vi "Display Tree Item.vi"(8 "error in (no error)":errorcluster, 10 "Tag":string, 11 "Application Data in":T1) -> (0 "error out":errorcluster, 3 "Application Data out":T1)   [LabVIEW 2017, in "DSF Mini Explorer.lvlib"]
uses:
  DSF Mini Explorer.lvlib
  Application Data.ctl
  VeriStand/Data Sharing Custom Device/Source/DSF Core.lvlibp/Classes/Configuration/Configuration Session.lvclass
  View Mode.ctl
  VeriStand/Data Sharing Custom Device/Source/DSF Core.lvlibp/Classes/Configuration/Read Plugin.vi
  VeriStand/Data Sharing Custom Device/Source/DSF Core.lvlibp/Classes/Configuration/Read Settings.vi
  VeriStand/Data Sharing Custom Device/Source/DSF Core.lvlibp/Classes/Configuration/Read Channel.vi
  VeriStand/Data Sharing Custom Device/Source/DSF Core.lvlibp/Classes/Configuration/Read Transfer.vi
  VeriStand/Data Sharing Custom Device/Source/DSF Core.lvlibp/Classes/Configuration/Read Group.vi
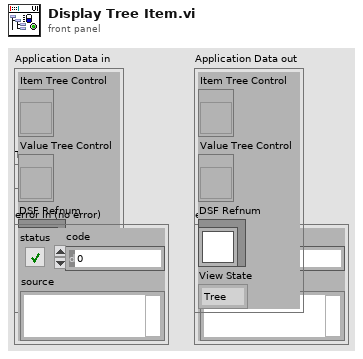
[diagram p1: front panel]
types:
  T1 = typedef "DSF Mini Explorer.lvlib/Application Data.ctl" = cluster{"Item Tree Control":refnum<vi>, "Value Tree Control":refnum<vi>, "DSF Refnum":refnum<class "Configuration Session.lvclass">, "View State":T2}
  T2 = typedef "DSF Mini Explorer.lvlib/View Mode.ctl" = enum16{"Tree", "List"}
  T3 = typedef "DSF Core.lvlibp/DSF Version Info.ctl" = cluster{"major":u32, "minor":u32, "fix":u32, "build":string}
  T4 = typedef "DSF Mini Explorer.lvlib/Tree Item Type.ctl" = enum16{"Plugin", "Group", "Transfer", "Channel", "Setting"}
  T5 = typedef "DSF Core.lvlibp/DSF Group Info.ctl" = cluster{"direction":T6, "timing":T7, "transfer ids":string[], "settings id":string, "thread":i32, "timeout behavior":T8}
  T6 = typedef "DSF Core.lvlibp/DSF Direction.ctl" = enum8{"Tx", "Rx"}
  T7 = typedef "DSF Core.lvlibp/DSF Timing Info.ctl" = cluster{"priority":u64, "decimation":u64, "offset":u64}
  T8 = typedef "DSF Core.lvlibp/DSF Timeout Behavior.ctl" = enum8{"Increment Late Count", "Throw Error"}
  T9 = typedef "DSF Core.lvlibp/DSF Transfer Info.ctl" = cluster{"byte order":T10, "channel ids":string[], "settings id":string}
  T10 = typedef "DSF Core.lvlibp/DSF Byte Order.ctl" = enum8{"big-endian", "little-endian"}
  T11 = typedef "DSF Core.lvlibp/DSF Channel Info.ctl" = cluster{"string buffer offset":u64, "string data type":T12, "engine data type":T12, "settings id":string, "units":string}
  T12 = typedef "DSF Core.lvlibp/DSF Data Type.ctl" = enum8{"Bool", "SGL", "DBL", "I8", "I16", "I32", "I64", "U8", "U16", "U32", "U64"}
  T13 = typedef "DSF Core.lvlibp/DSF Settings Info.ctl" = cluster{"key":string, "value":string}[]
  T14 = typedef "DSF Core.lvlibp/DSF Plugin Info.ctl" = cluster{"components":string[], "timing":T7, "group ids":string[], "settings id":string, "threads":T15[]}
  T15 = typedef "DSF Core.lvlibp/DSF Engine Plugin Thread Configuration.ctl" = cluster{"buffer converter settings":T13, "transceiver settings":T13, "custom settings":T13, "processor":i32, "priority offset":i16}
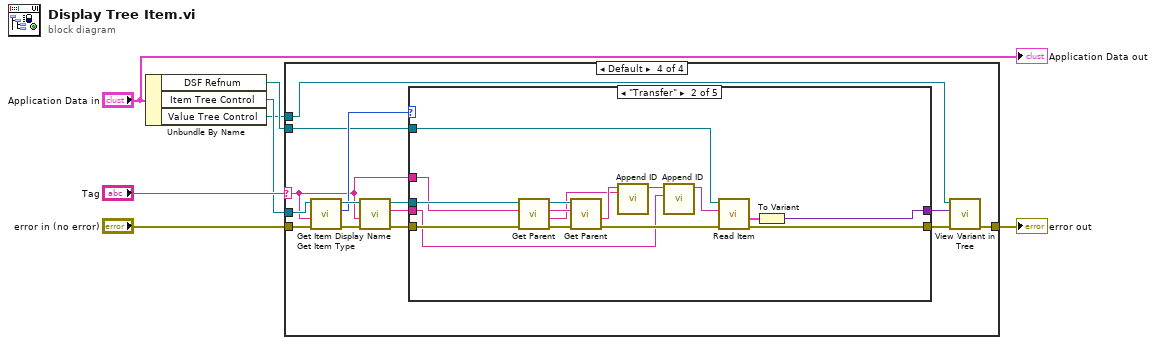
[diagram p0: block diagram]
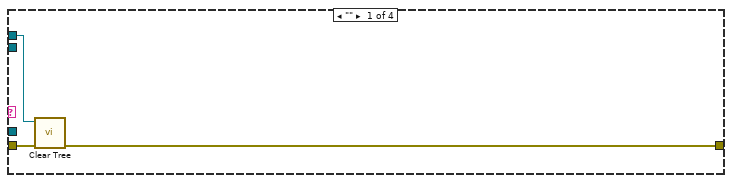
[diagram p2: hidden frame]
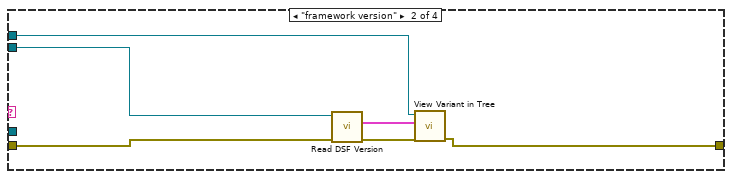
[diagram p3: hidden frame]
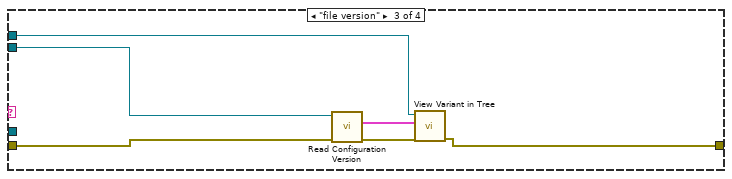
[diagram p4: hidden frame]
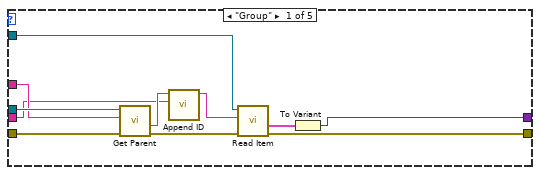
[diagram p5: hidden frame]
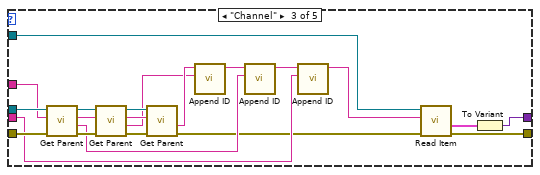
[diagram p6: hidden frame]
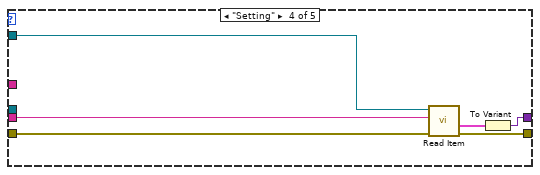
[diagram p7: hidden frame]
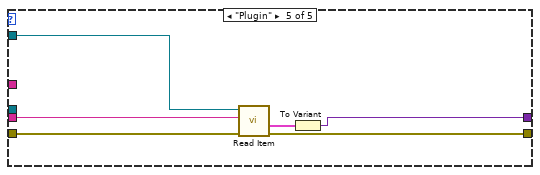
[diagram p8: hidden frame]
diagram:
  n1 = Unbundle By Name("Application Data in") -> ("DSF Refnum"=w5:refnum<class "Configuration Session.lvclass">, "Item Tree Control"=w4:refnum<vi>, "Value Tree Control"=w2:refnum<vi>)
  n2 = case shown="Default" "Tag" {
    selector: "Tag" -> [_ _ _ w24]
    tunnel: w5 -> [_ w16 w22 w31]
    tunnel: w4 -> [_ _ _ w30]
    tunnel: "error in (no error)" -> [w10 w15 w21 w29]
    tunnel: w2 -> [w8 w11 w17 w26]
    tunnel: [w9 w13 w19 w25] -> w1
    frame "" {
      n3 = call "Clear Tree.vi"("error in (no error)"=w10, "TreeControl in"=w8) -> ("error out"=w9:errorcluster)  [unwired: 9 in]
    }
    frame "framework version" {
      n4 = call "Read DSF Version.vi"("error in (no error)"=w15, "Configuration Session in"=w16) -> ("error out"=w14:errorcluster, "dsfversion"=w12:T3)  [unwired: 7 in, 1 out]
      n5 = call "View Variant in Tree.vi"("error in (no error)"=w14, "Variant"=w12, "TreeControl in"=w11) -> ("error out"=w13:errorcluster)  [unwired: 8 in]
    }
    frame "file version" {
      n6 = call "Read Configuration Version.vi"("error in (no error)"=w21, "Configuration Session in"=w22) -> ("error out"=w20:errorcluster, "version"=w18:T3)  [unwired: 7 in, 1 out]
      n7 = call "View Variant in Tree.vi"("error in (no error)"=w20, "Variant"=w18, "TreeControl in"=w17) -> ("error out"=w19:errorcluster)  [unwired: 8 in]
    }
    frame Default {
      n8 = call "Get Item Type.vi"("error in (no error)"=w29, "Tag"=w24, "TreeControl in"=w30) -> ("error out"=w35:errorcluster, "Item Type"=w33:T4, "TreeControl out"=w34:refnum<vi>)  [unwired: 6 in]
      n9 = call "Get Item Display Name.vi"("error in (no error)"=w35, "Tag"=w24, "TreeControl in"=w34) -> ("error out"=w36:errorcluster, "display name"=w32:string, "TreeControl out"=w23:refnum<vi>)  [unwired: 6 in]
      n10 = case shown="\"Transfer\"" w33 {
        tunnel: w32 -> [w39 w48 w67 w85 w91]
        tunnel: [w46 w62 w83 w90 w95] -> w28
        tunnel: w36 -> [w42 w59 w78 w86 w96]
        tunnel: w31 -> [w44 w61 w81 w87 w94]
        tunnel: [w45 w60 w82 w88 w93] -> w27
        tunnel: w24 -> [w41 w56 w76 _ _]
        tunnel: w23 -> [w43 w58 w77 _ _]
        frame "Group" {
          n11 = call "Get Parent.vi"("error in (no error)"=w42, "tag"=w41, "TreeControl in"=w43) -> ("error out"=w38:errorcluster, "parent name"=w40:string)  [unwired: 5 in, 2 out]
          n12 = call "Append ID.vi"("name"=w39, "initial id string (\"\")"=w40) -> ("appended id string"=w37:string)  [unwired: 9 in]
          n13 = call-poly "Read Item.vi"("error in (no error)"=w38, "Group ID"=w37, "Configuration Session in"=w44) -> ("error out"=w46:errorcluster, "value"=w47:T5)  [unwired: 5 in, 2 out]
          n14 = To Variant(anything=w47) -> (Variant=w45:variant)
        }
        frame "Transfer" {
          n15 = call "Get Parent.vi"("error in (no error)"=w59, "tag"=w56, "TreeControl in"=w58) -> ("error out"=w54:errorcluster, "parent name"=w51:string, "parent tag"=w53:string, "TreeControl out"=w55:refnum<vi>)  [unwired: 5 in]
          n16 = call "Get Parent.vi"("error in (no error)"=w54, "tag"=w53, "TreeControl in"=w55) -> ("error out"=w50:errorcluster, "parent name"=w52:string)  [unwired: 5 in, 2 out]
          n17 = call "Append ID.vi"("name"=w51, "initial id string (\"\")"=w52) -> ("appended id string"=w49:string)  [unwired: 9 in]
          n18 = call "Append ID.vi"("name"=w48, "initial id string (\"\")"=w49) -> ("appended id string"=w57:string)  [unwired: 9 in]
          n19 = call-poly "Read Item.vi"("error in (no error)"=w50, "Transfer ID"=w57, "Configuration Session in"=w61) -> ("error out"=w62:errorcluster, "value"=w63:T9)  [unwired: 5 in, 2 out]
          n20 = To Variant(anything=w63) -> (Variant=w60:variant)
        }
        frame "Channel" {
          n21 = call "Get Parent.vi"("error in (no error)"=w78, "tag"=w76, "TreeControl in"=w77) -> ("error out"=w80:errorcluster, "parent name"=w69:string, "parent tag"=w79:string, "TreeControl out"=w64:refnum<vi>)  [unwired: 5 in]
          n22 = call "Get Parent.vi"("error in (no error)"=w80, "tag"=w79, "TreeControl in"=w64) -> ("error out"=w74:errorcluster, "parent name"=w71:string, "parent tag"=w73:string, "TreeControl out"=w75:refnum<vi>)  [unwired: 5 in]
          n23 = call "Get Parent.vi"("error in (no error)"=w74, "tag"=w73, "TreeControl in"=w75) -> ("error out"=w65:errorcluster, "parent name"=w72:string)  [unwired: 5 in, 2 out]
          n24 = call "Append ID.vi"("name"=w71, "initial id string (\"\")"=w72) -> ("appended id string"=w70:string)  [unwired: 9 in]
          n25 = call "Append ID.vi"("name"=w69, "initial id string (\"\")"=w70) -> ("appended id string"=w68:string)  [unwired: 9 in]
          n26 = call "Append ID.vi"("name"=w67, "initial id string (\"\")"=w68) -> ("appended id string"=w66:string)  [unwired: 9 in]
          n27 = call-poly "Read Item.vi"("error in (no error)"=w65, "Channel ID"=w66, "Configuration Session in"=w81) -> ("error out"=w83:errorcluster, "value"=w84:T11)  [unwired: 5 in, 2 out]
          n28 = To Variant(anything=w84) -> (Variant=w82:variant)
        }
        frame "Setting" {
          n29 = call-poly "Read Item.vi"("error in (no error)"=w86, "Settings ID"=w85, "Configuration Session in"=w87) -> ("error out"=w90:errorcluster, "value"=w89:T13)  [unwired: 5 in, 2 out]
          n30 = To Variant(anything=w89) -> (Variant=w88:variant)
        }
        frame "Plugin" {
          n31 = call-poly "Read Item.vi"("error in (no error)"=w96, "Plugin ID"=w91, "Configuration Session in"=w94) -> ("error out"=w95:errorcluster, "value"=w92:T14)  [unwired: 5 in, 2 out]
          n32 = To Variant(anything=w92) -> (Variant=w93:variant)
        }
      }
      n33 = call "View Variant in Tree.vi"("error in (no error)"=w28, "Variant"=w27, "TreeControl in"=w26) -> ("error out"=w25:errorcluster)  [unwired: 8 in]
    }
  }
  "error out" <- w1
  "Application Data out" <- "Application Data in"
